vi "close.vi"(8 "error in":errorcluster, 11 "Shared Library Module runtime in":refnum<class "Shared Library Module runtime.lvclass">) -> (0 "error out":errorcluster)   [LabVIEW 2013, in "Shared Library Module runtime.lvclass"]
doc: "Provides an interface for terminating a module instance. While this interface performs no operations, a child should close and deallocate any open references or memory.Platypus Framework 1.0.1.60\nNI Systems Engineering - National Instruments"
uses:
  Shared Library Module runtime.lvclass
  Shared Library Module runtime.lvclass/Shared Library Module runtime.ctl
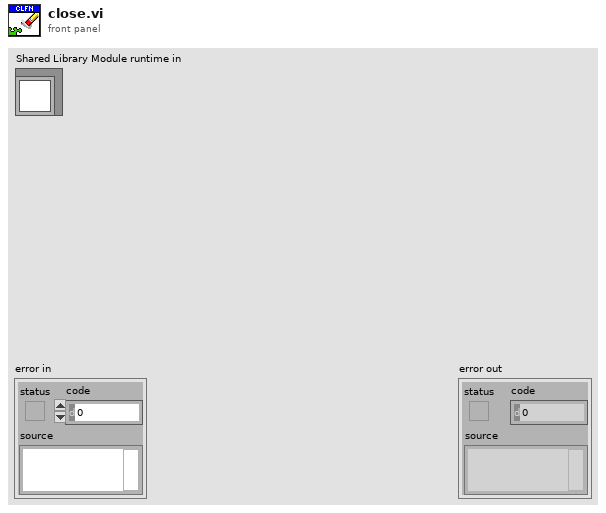
[diagram p1: front panel]
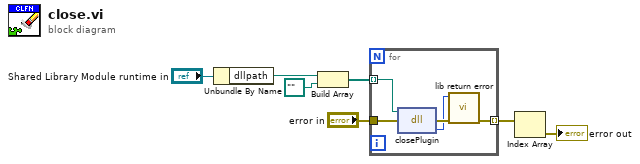
[diagram p0: block diagram]
diagram:
  n1 = Unbundle By Name("Shared Library Module runtime in") -> ("dllpath"=w7:path)
  n2 = Build Array(w7, path "" ("element")) -> (w5:path[])
  n3 = for {
    tunnel: "error in" -> [w12]
    tunnel: w5 -> [w11] mode=indexing
    tunnel: [w8] -> w4 mode=indexing
    n4 = dll-call lib="?" fn="closePlugin"(path in=w11, error in=w12) -> (error out=w10:errorcluster, "return type"=w9:i32)  [unwired: 1 in, 1 out]
    n5 = call "lib return error.vi"("error in"=w10, "return value"=w9) -> ("error out"=w8:errorcluster)  [unwired: 9 in]
  }
  n6 = Index Array(array=w4) -> (element=→"error out":errorcluster)  [unwired: 1 in]
